vi "Lezeti_Power_Monitor_21_d.vi"() -> ()   [LabVIEW 2014]
uses:
  <vilib>/measure/NI_MAPro.lvlib
  <vilib>/measure/madcrms.llb/Basic Averaged DC-RMS for N Chan.vi
  <vilib>/measure/madcrms.llb/Basic Averaged DC-RMS for 1 Chan.vi
  <vilib>/Utility/file.llb/Write To Spreadsheet File (DBL).vi
panel:
  in  "High Resolution Waveform Data Path":path
  out "Power Factor":dbl
  in  "Average Power Output File":path
  out "Run Date":string
  out "Run Time":string
  out "Elapsed Time (s)":dbl
  out "Apparent Power (VA)":dbl
  out "Average Power (Watts)":dbl
  out "Instantaneous Power Waveform":waveform(dbl)[](graph)
  out "RMS Voltage L-N":dbl
  out "L2 RMS Current":dbl
  out "L1 RMS Current":dbl
  in  "Burden Resistor (ohms) (1000)":dbl
  in  "CT Ratio (Iout/Iin) (.0003332)":dbl
  in  "Acquire Sample Size (1000)":dbl
  in  "Acquire Rate (Hz) (1000)":dbl
  in  "Acquire Timeout (1000)":dbl
  out "Line 2 Current Waveform":waveform(dbl)[](graph)
  out "Line 1 Current Waveform":waveform(dbl)[](graph)
  out "Voltage L-N":waveform(dbl)[](graph)
  in  "stop":bool
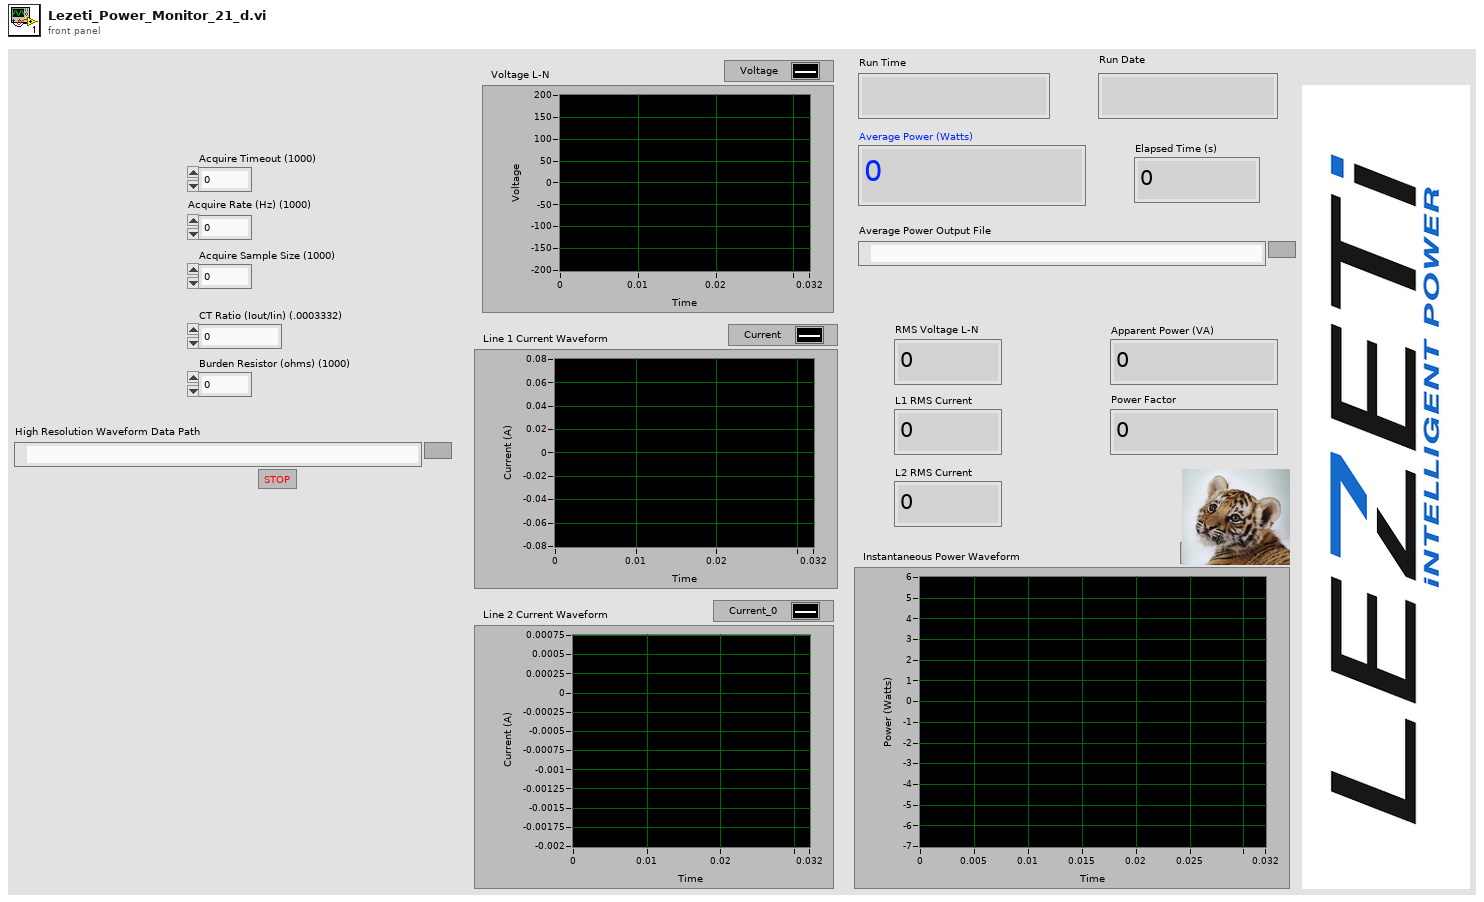
[diagram p1: front panel]
types:
  T1 = typedef "NI_Matrix.lvlib/RealMatrix.ctl" = dbl[][]
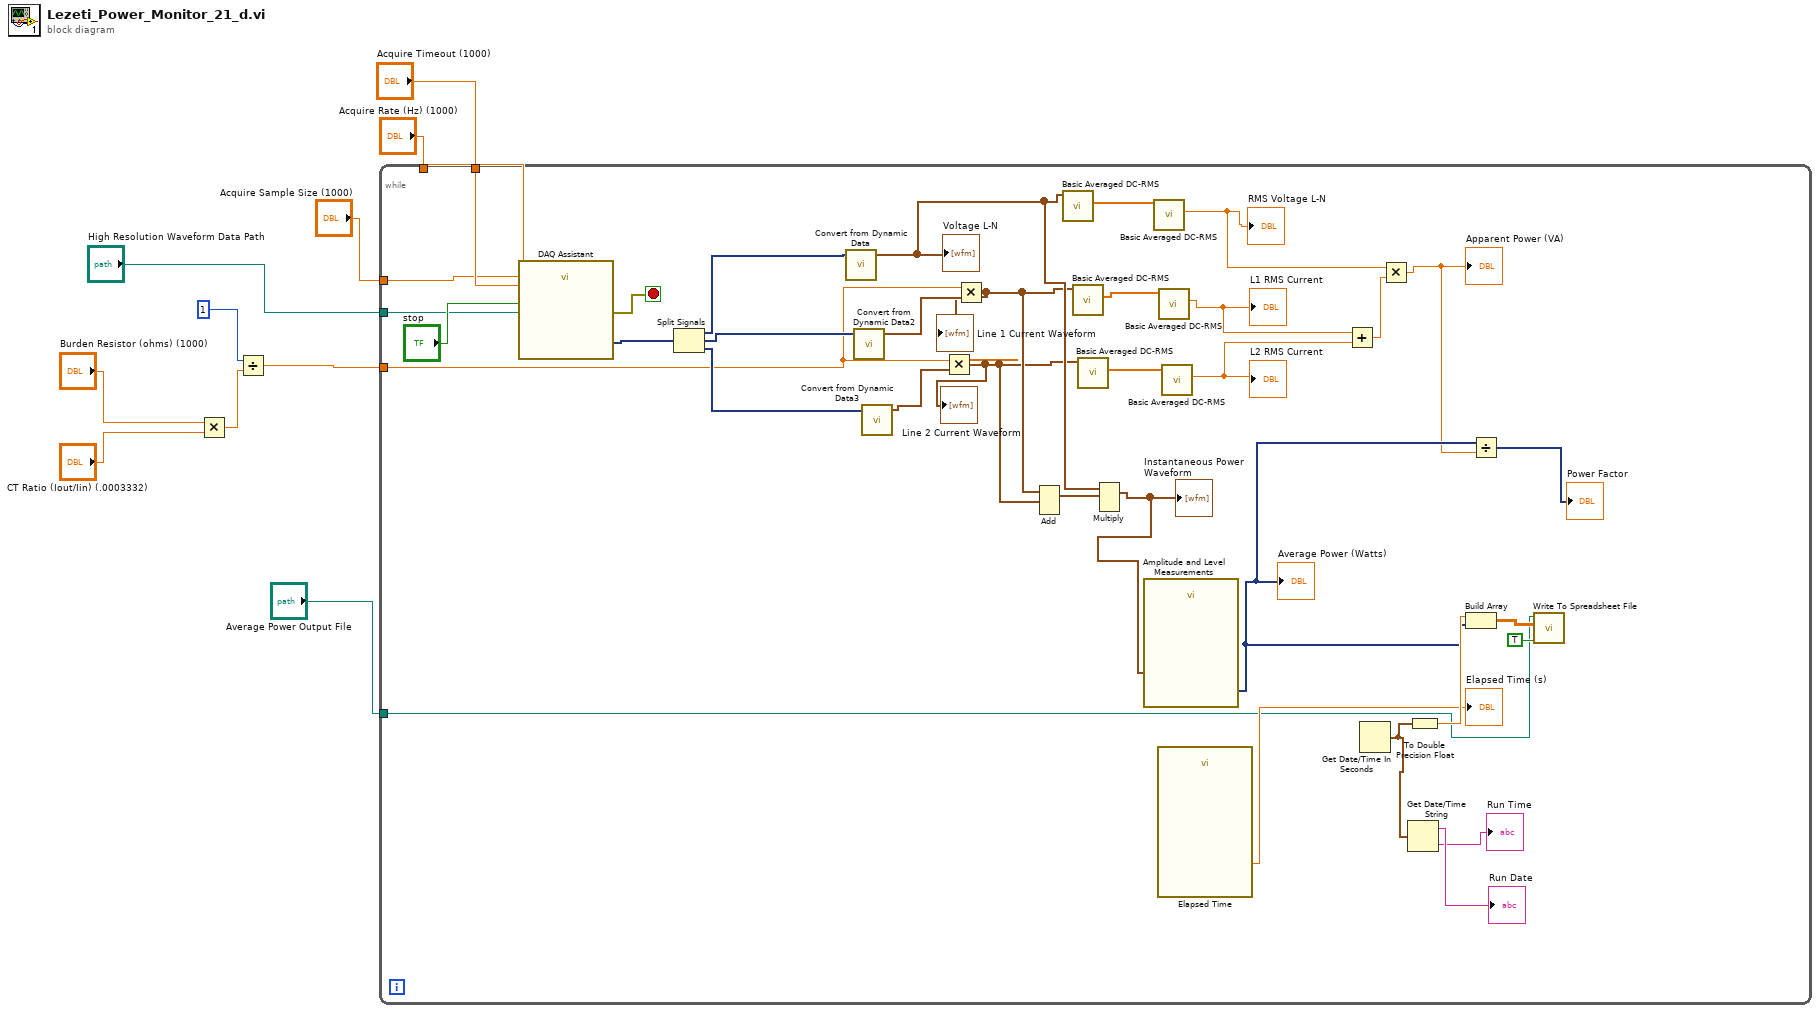
[diagram p0: block diagram]
diagram:
  n1 = Multiply(x="Burden Resistor (ohms) (1000)", y="CT Ratio (Iout/Iin) (.0003332)") -> (x*y=w4:dbl)
  n2 = Divide(x=1, y=w4) -> (x/y=w3:dbl)
  n3 = while {
    tunnel: "Acquire Timeout (1000)" -> [w42]
    tunnel: "Acquire Rate (Hz) (1000)" -> [w36]
    tunnel: "Acquire Sample Size (1000)" -> [w35]
    tunnel: w3 -> [w34]
    tunnel: "Average Power Output File" -> [w15]
    tunnel: "High Resolution Waveform Data Path" -> [w11]
    stop <- w37 stop-if-true
    n4 = call "DAQ Assistant"(2:w36, 3:w35, "timeout (s)"=w42, "stop (F)"="stop", "file path"=w11) -> ("data"=w46:dynamicdata, "error out"=w37:errorcluster)  [unwired: 11 in, 2 out]
    n5 = Split Signals(w46) -> (w45:dynamicdata, w44:dynamicdata, w43:dynamicdata)  [unwired: 3 in]
    n6 = call "Convert from Dynamic Data"("Dynamic Data Type"=w45) -> ("Array of Waveform"=w31:waveform(dbl)[])  [unwired: 3 in]
    "Voltage L-N" <- w31
    n7 = call "Convert from Dynamic Data2"("Dynamic Data Type"=w44) -> ("Array of Waveform"=w33:waveform(dbl)[])  [unwired: 3 in]
    n8 = call "Convert from Dynamic Data3"("Dynamic Data Type"=w43) -> ("Array of Waveform"=w32:waveform(dbl)[])  [unwired: 3 in]
    n9 = Multiply(x=w34, y=w32) -> (x*y=w27:waveform(dbl)[])
    "Line 2 Current Waveform" <- w27
    n10 = Multiply(x=w34, y=w33) -> (x*y=w28:waveform(dbl)[])
    "Line 1 Current Waveform" <- w28
    n11 = Add(1:w27, 2:w28) -> (0:w30:waveform(dbl)[])  [unwired: 1 in, 1 out]
    n12 = call-poly <vilib>:"Basic Averaged DC-RMS.vi"("signals in"=w31) -> ("RMS values"=w40:dbl[])  [unwired: 7 in, 3 out]
    n13 = call-poly <vilib>:"Basic Averaged DC-RMS.vi"("signals in"=w28) -> ("RMS values"=w39:dbl[])  [unwired: 7 in, 3 out]
    n14 = call-poly <vilib>:"Basic Averaged DC-RMS.vi"("signals in"=w27) -> ("RMS values"=w38:dbl[])  [unwired: 7 in, 3 out]
    n15 = Multiply(1:w30, 2:w31) -> (0:w29:waveform(dbl)[])  [unwired: 1 in, 1 out]
    "Instantaneous Power Waveform" <- w29
    n16 = call "Amplitude and Level Measurements"("Signals"=w29) -> ("Mean (DC)"=w14:dynamicdata)  [unwired: 13 in, 1 out]
    "Average Power (Watts)" <- w14
    n17 = call-poly <vilib>:"Basic Averaged DC-RMS.vi"("signal in"=w40) -> ("RMS value"=w23:dbl)  [unwired: 7 in, 3 out]
    "RMS Voltage L-N" <- w23
    n18 = call "Elapsed Time"() -> ("Elapsed Time (s)"=→"Elapsed Time (s)":dbl)  [unwired: 12 in, 7 out]
    n19 = call-poly <vilib>:"Basic Averaged DC-RMS.vi"("signal in"=w39) -> ("RMS value"=w26:dbl)  [unwired: 7 in, 3 out]
    "L1 RMS Current" <- w26
    n20 = call-poly <vilib>:"Basic Averaged DC-RMS.vi"("signal in"=w38) -> ("RMS value"=w25:dbl)  [unwired: 7 in, 3 out]
    "L2 RMS Current" <- w25
    n21 = Add(x=w26, y=w25) -> (x+y=w24:dbl)
    n22 = Get Date/Time In Seconds() -> (seconds since 1Jan1904=w19:timestamp)
    n23 = Multiply(x=w23, y=w24) -> (x*y=w13:dbl)
    "Apparent Power (VA)" <- w13
    n24 = Get Date/Time String(seconds (now)=w19) -> (date string=→"Run Date":string, time string=→"Run Time":string)  [unwired: 2 in]
    n25 = To Double Precision Float(number=w19) -> (double precision float=w20:dbl)
    n26 = Build Array(w20, w14) -> (w21:T1)
    n27 = Divide(x=w14, y=w13) -> (x/y=→"Power Factor":dynamicdata)
    n28 = call-poly <vilib>:"Write To Spreadsheet File.vi"("append to file? (new file:F)"=TRUE, "2D data"=w21, "file path (dialog if empty)"=w15) -> ()  [unwired: 5 in, 1 out]
  }
